vi "Begin.vi"   [LabVIEW 2019, in "LabPack.lvlib" / "Writer.lvclass"]
doc: "Starts the internal encoder. This is required to be called before any other encoding VIs are used."
uses:
  Writer.lvclass
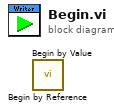
[diagram p0: block diagram]
diagram:
  n1 = call "Begin by Reference.vi"() -> ()  [unwired: 10 in, 2 out]
  n2 = call "Begin by Value.vi"() -> ()  [unwired: 10 in, 2 out]
